vi "Query Questionable Status Register.vi"(8 "error in (no error)":errorcluster, 11 "VISA resource name":refnum<visa-resource-name>) -> (0 "error out":errorcluster, 1 "Questionable Data Message":string, 3 "VISA resource name out":refnum<visa-resource-name>)   [LabVIEW 2019, in "Agilent 681x Series.lvlib"]
doc: "Queries the event register for the Questionable Status Register group. Essentially, it is used to observe possible invalid results. For example, if any of the protections are tripped, the questionable status register will be set. This VI will then return the corresponding warning(s)."
uses:
  <instrlib>/Agilent 681x Series/Agilent 681x Series.lvlib
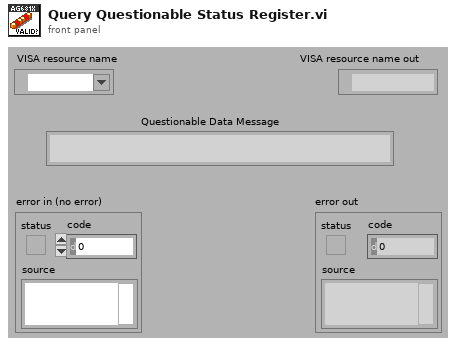
[diagram p1: front panel]
types:
  T1 = cluster{"Boolean array[0]":bool, "Boolean array[1]":bool, "Boolean array[2]":bool, "Boolean array[3]":bool, "Boolean array[4]":bool, "Boolean array[5]":bool, "Boolean array[6]":bool, "Boolean array[7]":bool, "Boolean array[8]":bool, "Boolean array[9]":bool, "Boolean array[10]":bool, "Boolean array[11]":bool, "Boolean array[12]":bool, "Boolean array[13]":bool, "Boolean array[14]":bool, "Boolean array[15]":bool}
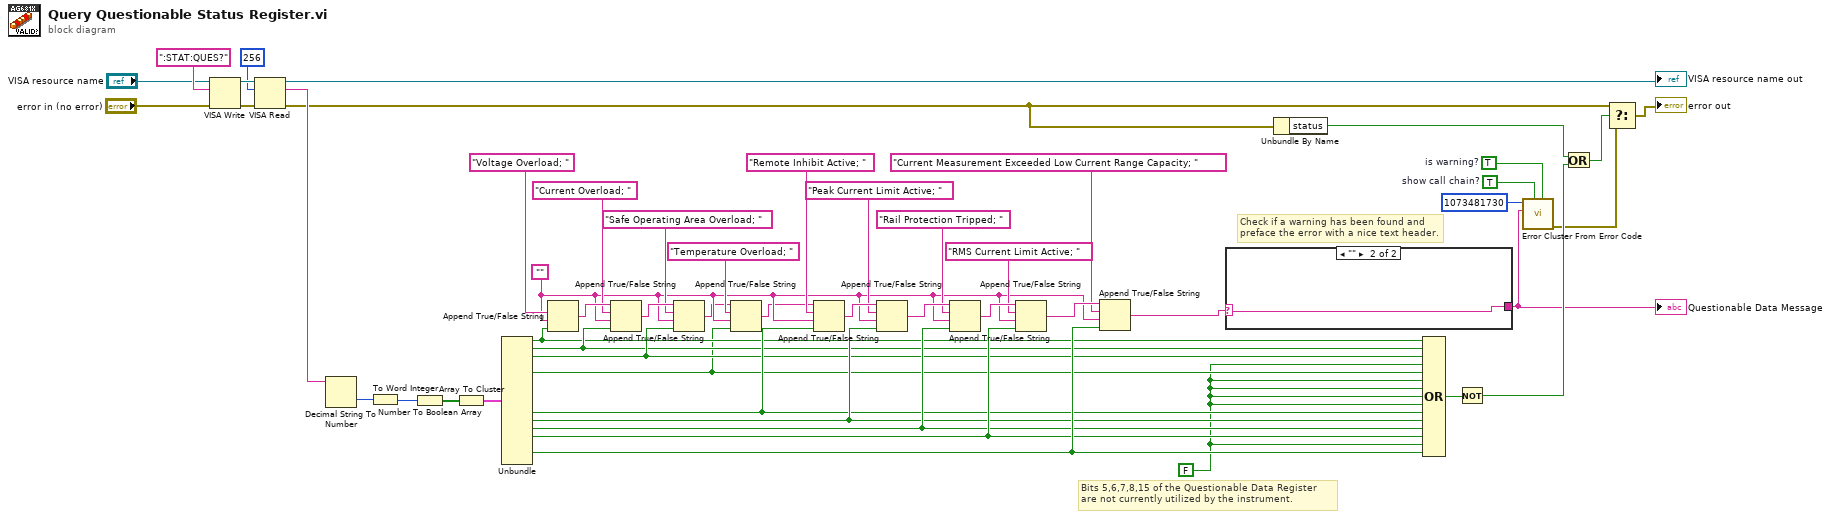
[diagram p0: block diagram]
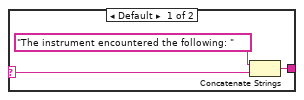
[diagram p2: hidden frame]
diagram:
  w8 = TRUE  # is warning?
  w9 = TRUE  # show call chain?
  w1 = FALSE
  w28 = ""
  # "Check if a warning has been found and preface the error with a nice text header."
  # "Bits 5,6,7,8,15 of the Questionable Data Register are not currently utilized by the instrument."
  n1 = VISA Write(VISA resource name="VISA resource name", write buffer=":STAT:QUES?", error in (no error)="error in (no error)") -> (VISA resource name out=w50:refnum<visa-resource-name>, error out=w51:errorcluster)  [unwired: 1 out]
  n2 = VISA Read(VISA resource name=w50, byte count=u32 256, error in (no error)=w51) -> (VISA resource name out=→"VISA resource name out":refnum<visa-resource-name>, read buffer=w48:string, error out=w12:errorcluster)  [unwired: 1 out]
  n3 = Decimal String To Number(string=w48) -> (number=w45:i32)  [unwired: 2 in, 1 out]
  n4 = To Word Integer(number=w45) -> (16bit integer=w46:i16)
  n5 = Number To Boolean Array(number=w46) -> (Boolean array=w47:bool[])
  n6 = Array To Cluster(array=w47) -> (cluster=w44:T1)
  n7 = Unbundle(w44) -> ("Boolean array[0]"=w18:bool, "Boolean array[1]"=w19:bool, "Boolean array[2]"=w20:bool, "Boolean array[4]"=w4:bool, "Boolean array[9]"=w21:bool, "Boolean array[10]"=w22:bool, "Boolean array[11]"=w23:bool, "Boolean array[12]"=w24:bool, "Boolean array[14]"=w25:bool)  [unwired: 7 out]
  n8 = Append True/False String(1:w18, 2:w28, 3:"Voltage Overload; " ("true string")) -> (0:w43:string)  [unwired: 1 in]
  n9 = Append True/False String(1:w19, 2:w28, 3:"Current Overload; " ("true string"), 4:w43) -> (0:w42:string)
  n10 = Append True/False String(1:w20, 2:w28, 3:"Safe Operating Area Overload; " ("true string"), 4:w42) -> (0:w3:string)
  n11 = Append True/False String(1:w4, 2:w28, 3:"Temperature Overload; " ("true string"), 4:w3) -> (0:w2:string)
  n12 = Append True/False String(1:w21, 2:w28, 3:"Remote Inhibit Active; " ("true string"), 4:w2) -> (0:w41:string)
  n13 = Append True/False String(1:w22, 2:w28, 3:"Peak Current Limit Active; " ("true string"), 4:w41) -> (0:w40:string)
  n14 = Append True/False String(1:w23, 2:w28, 3:"Rail Protection Tripped; " ("true string"), 4:w40) -> (0:w39:string)
  n15 = Append True/False String(1:w24, 2:w28, 3:"RMS Current Limit Active; " ("true string"), 4:w39) -> (0:w38:string)
  n16 = Append True/False String(1:w25, 2:w28, 3:"Current Measurement Exceeded Low Current Range Capacity; " ("true string"), 4:w38) -> (0:w6:string)
  n17 = case shown="\"\"" w6 {
    selector: w6 -> [w54 w56]
    tunnel: [w53 w56] -> w5
    frame Default {
      n18 = Concatenate Strings("The instrument encountered the following: " ("true string"), w54) -> (w53:string)
    }
    frame "" {
    }
  }
  "Questionable Data Message" <- w5
  n19 = Unbundle By Name(w12) -> ("status"=w15:bool)
  n20 = Compound Arithmetic op=OR(w18, w19, w20, w1, w4, w1, w1, w1, w1, w21, w22, w23, w24, w1, w25) -> (w17:bool)
  n21 = Not(x=w17) -> (.not. x?=w16:bool)
  n22 = call <vilib>:"Error Cluster From Error Code.vi"("is warning? (False)"=w8, "show call chain? (False)"=w9, "error message (\"\")"=w5, "error code (0)"=1073481730 ("t")) -> ("error out"=w11:errorcluster)  [unwired: 5 in]
  n23 = Or(x=w15, y=w16) -> (x .or. y?=w14:bool)
  n24 = Select(t=w12, s=w14, f=w11) -> (s? t:f=→"error out":errorcluster)
